vi "Image to array.vi"() -> ()   [LabVIEW 2021]
panel:
  out "Image Pixels (Float)":sgl[][](array[numeric])
  out "Image":T1(plugin-control)
  in  "File Path":path
  in  "Image Type":T2 items=["Grayscale (U8)", "Grayscale (I16)", "Grayscale (SGL)", "Complex (CSG)", "RGB (U32)", "HSL (U32)", "RGB (U64)", "Grayscale (U16)"]
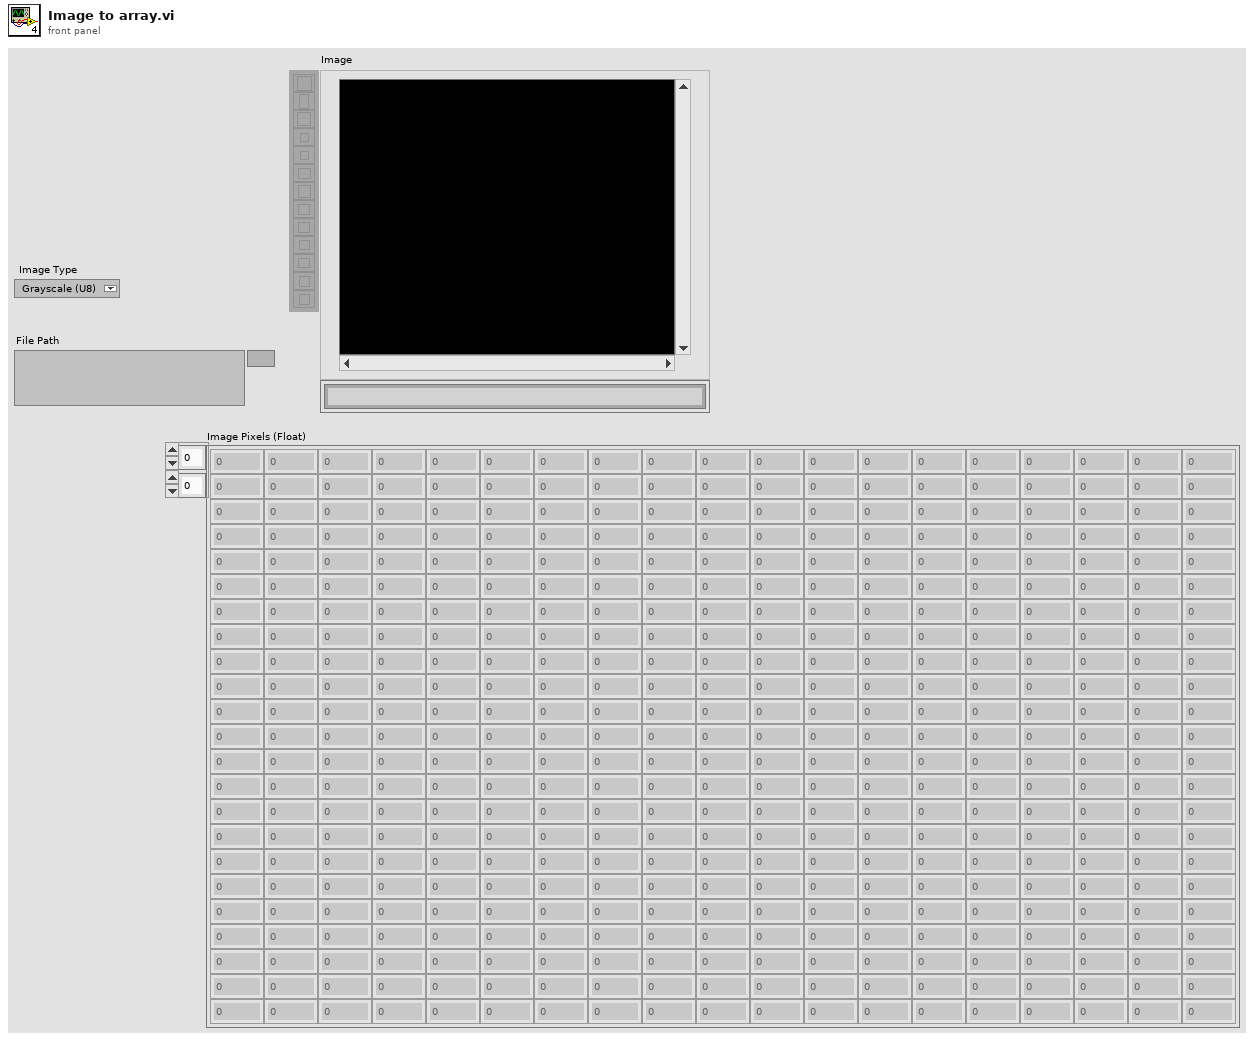
[diagram p1: front panel]
types:
  T1 = typedef "IMAQ Image.ctl" = refnum<image>
  T2 = typedef "Image Type" = u32
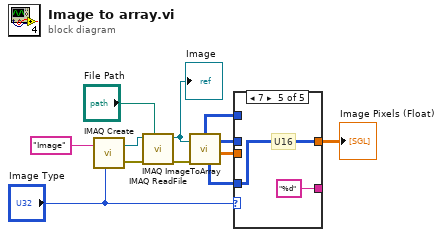
[diagram p0: block diagram]
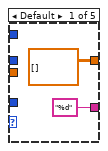
[diagram p2: hidden frame]
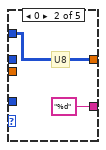
[diagram p3: hidden frame]
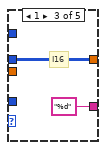
[diagram p4: hidden frame]
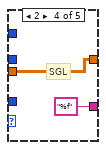
[diagram p5: hidden frame]
diagram:
  n1 = call "IMAQ Create"("Image Name"="Image", "Image Type"="Image Type") -> ("New Image"=w10:T1, "error out"=w11:errorcluster)  [unwired: 3 in]
  n2 = call "IMAQ ReadFile"("File Path"="File Path", "error in (no error)"=w11, "Image"=w10) -> ("error out"=w1:errorcluster, "Image Out"=w2:T1)  [unwired: 4 in, 3 out]
  "Image" <- w2
  n3 = call "IMAQ ImageToArray"("error in (no error)"=w1, "Image"=w2) -> ("Image Pixels (U16)"=w4:u16[][], "Image Pixels (Float)"=w5:sgl[][], "Image Pixels (U8)"=w6:u8[][], "Image Pixels (I16)"=w8:i16[][])  [unwired: 2 in, 1 out]
  n4 = case shown="7" "Image Type" {
    tunnel: w8 -> [_ _ w17 _ _]
    tunnel: w6 -> [_ w16 _ _ _]
    tunnel: w5 -> [_ _ _ w19 _]
    tunnel: w4 -> [_ _ _ _ w21]
    tunnel: [sgl[][] [] ("Image Pixels (Float)") w16 w17 w19 w21] -> w3
    tunnel: ["%d" ("Format-String") "%d" ("Format-String") "%d" ("Format-String") "%f" ("Format-String") "%d" ("Format-String")] -> _
    frame Default {
    }
    frame 0 {
      # "U8"
    }
    frame 1 {
      # "I16"
    }
    frame 2 {
      # "SGL"
    }
    frame 7 {
      # "U16"
    }
  }
  "Image Pixels (Float)" <- w3
